vi "Client.vi"() -> ()   [LabVIEW 2009]
panel:
  in  "Example:":string(combo)
  out "time":string
  out "TCP_F":bool
  in  "Exit":bool
  out "IP-status":string
  in  "IP-address":string="10.3.1.41"
  in  "Result?":bool
  in  "Result":string
  in  "Status?":bool
  in  "Status":string
  in  "Send":bool
  in  "CMD":string="Set_PJVS"
  out "TCP_T":bool caption="Status TCP connection"
  out "connection ID":refnum<k5>
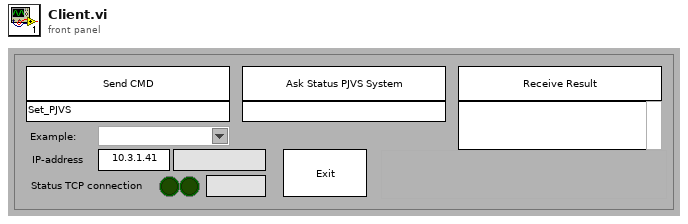
[diagram p1: front panel]
types:
  T1 = enum32{"invalid app kind", "Development System", "Run Time System", "Student Edition", "Embedded LabVIEW", "Evaluation", "Custom"}
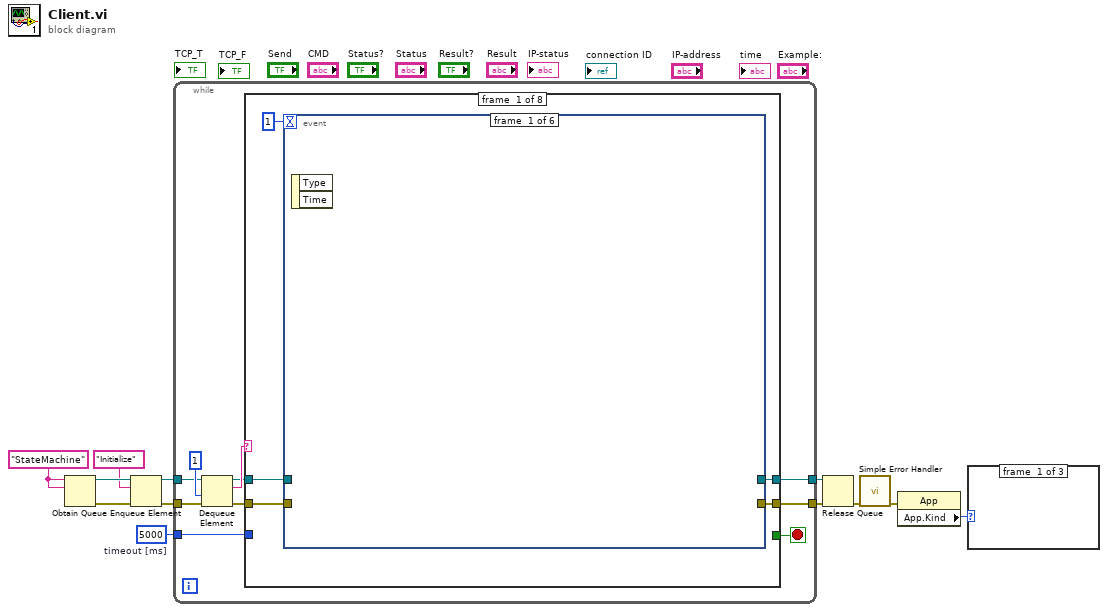
[diagram p0: block diagram]
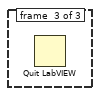
[diagram p3: hidden frame]
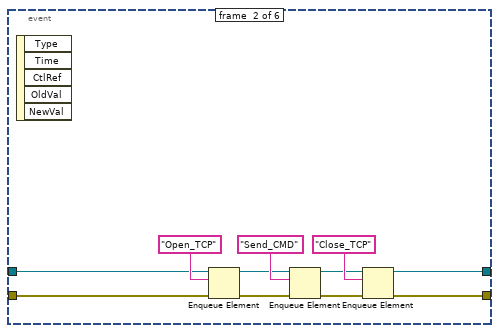
[diagram p4: hidden frame]
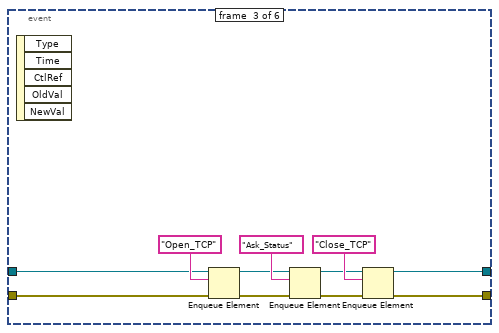
[diagram p5: hidden frame]
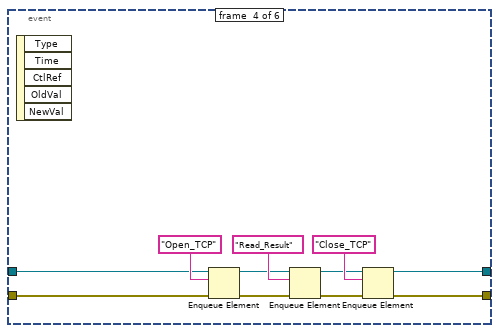
[diagram p6: hidden frame]
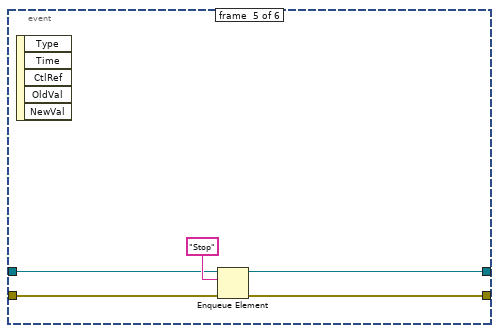
[diagram p7: hidden frame]
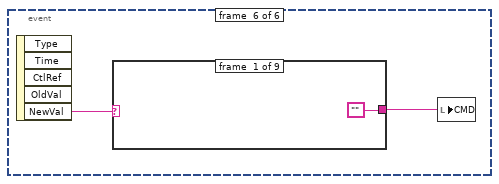
[diagram p8: hidden frame]
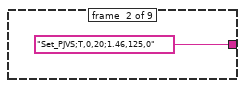
[diagram p9: hidden frame]
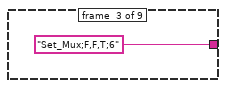
[diagram p10: hidden frame]
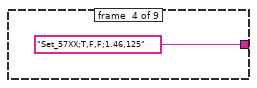
[diagram p11: hidden frame]
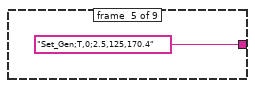
[diagram p12: hidden frame]
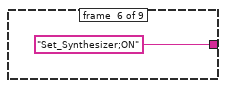
[diagram p13: hidden frame]
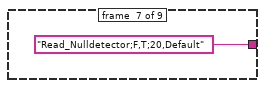
[diagram p14: hidden frame]
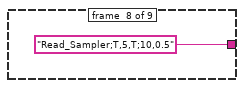
[diagram p15: hidden frame]
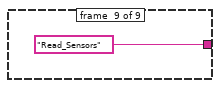
[diagram p16: hidden frame]
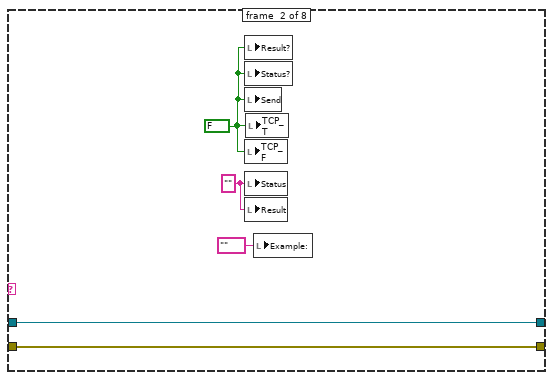
[diagram p17: hidden frame]
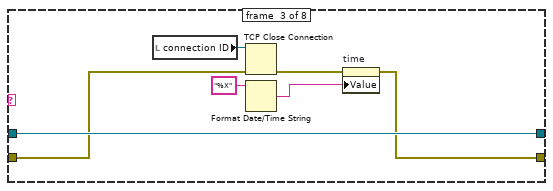
[diagram p18: hidden frame]
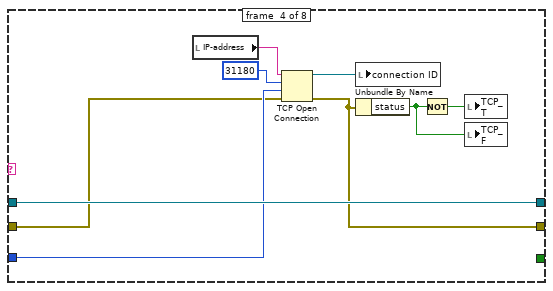
[diagram p19: hidden frame]
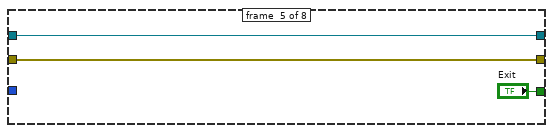
[diagram p20: hidden frame]
diagram:
  w2 = 5000  # timeout [ms]
  w9 = "StateMachine" ("element")
  n1 = Obtain Queue(name (unnamed)=w9, element data type=w9) -> (queue out=w12:refnum<queue>, error out=w11:errorcluster)  [unwired: 3 in, 1 out]
  n2 = Enqueue Element(queue=w12, element="Initialize", error in (no error)=w11) -> (queue out=w8:refnum<queue>, error out=w7:errorcluster)  [unwired: 1 in, 1 out]
  n3 = while {
    tunnel: w8 -> [w21]
    tunnel: w7 -> [w20]
    tunnel: [w18] -> w3
    tunnel: w2 -> [w15]
    tunnel: [w14] -> w1
    stop <- w13 stop-if-true
    n4 = Dequeue Element(queue=w21, timeout in ms (-1)=1, error in (no error)=w20) -> (queue out=w17:refnum<queue>, element=w19:string, error out=w16:errorcluster)  [unwired: 1 out]
    n5 = case shown="\"Read_Result\"" w19 {
      tunnel: [w24 w81 w88 w97 w100 w126 w148 w170] -> w18
      tunnel: w17 -> [w26 w81 w88 w97 w100 w126 w148 w170]
      tunnel: w16 -> [w25 w80 w86 w93 w98 w118 w144 w166]
      tunnel: w15 -> [_ _ _ w94 _ w108 w140 w162]
      tunnel: [w23 w80 w84 w92 w98 w101 w131 w153] -> w14
      tunnel: [_ _ _ _ "Exit" _ _ _] -> w13
      frame #0 {
        n6 = event shown="[5] \"Example:\": Value Change" {
          selector: _ -> [_ _ _ _ _ _]
          dyn-events: _ -> [_ _ _ _ _ _]
          timeout: 1 -> [_ _ _ _ _ _]
          tunnel: w26 -> [_ w31 w42 w53 w62 _]
          tunnel: w25 -> [_ w32 w43 w54 w61 _]
          tunnel: [_ w28 w39 w50 w64 _] -> w24
          tunnel: [_ w33 w44 w55 w63 _] -> w23
          event #0 {
            n7 = event-data() -> ()  [unwired: 1 in, 2 out]
          }
          event #1 {
            n8 = event-data() -> ()  [unwired: 1 in, 5 out]
            n9 = Enqueue Element(queue=w31, element="Open_TCP", error in (no error)=w32) -> (queue out=w30:refnum<queue>, error out=w35:errorcluster)  [unwired: 1 in, 1 out]
            n10 = Enqueue Element(queue=w30, element="Send_CMD", error in (no error)=w35) -> (queue out=w29:refnum<queue>, error out=w34:errorcluster)  [unwired: 1 in, 1 out]
            n11 = Enqueue Element(queue=w29, element="Close_TCP", error in (no error)=w34) -> (queue out=w28:refnum<queue>, error out=w33:errorcluster)  [unwired: 1 in, 1 out]
          }
          event #2 {
            n12 = event-data() -> ()  [unwired: 1 in, 5 out]
            n13 = Enqueue Element(queue=w42, element="Open_TCP", error in (no error)=w43) -> (queue out=w41:refnum<queue>, error out=w46:errorcluster)  [unwired: 1 in, 1 out]
            n14 = Enqueue Element(queue=w41, element="Ask_Status", error in (no error)=w46) -> (queue out=w40:refnum<queue>, error out=w45:errorcluster)  [unwired: 1 in, 1 out]
            n15 = Enqueue Element(queue=w40, element="Close_TCP", error in (no error)=w45) -> (queue out=w39:refnum<queue>, error out=w44:errorcluster)  [unwired: 1 in, 1 out]
          }
          event #3 {
            n16 = event-data() -> ()  [unwired: 1 in, 5 out]
            n17 = Enqueue Element(queue=w53, element="Open_TCP", error in (no error)=w54) -> (queue out=w52:refnum<queue>, error out=w57:errorcluster)  [unwired: 1 in, 1 out]
            n18 = Enqueue Element(queue=w52, element="Read_Result", error in (no error)=w57) -> (queue out=w51:refnum<queue>, error out=w56:errorcluster)  [unwired: 1 in, 1 out]
            n19 = Enqueue Element(queue=w51, element="Close_TCP", error in (no error)=w56) -> (queue out=w50:refnum<queue>, error out=w55:errorcluster)  [unwired: 1 in, 1 out]
          }
          event #4 {
            n20 = event-data() -> ()  [unwired: 1 in, 5 out]
            n21 = Enqueue Element(queue=w62, element="Stop", error in (no error)=w61) -> (queue out=w64:refnum<queue>, error out=w63:errorcluster)  [unwired: 1 in, 1 out]
          }
          event #5 {
            n22 = event-data() -> ("NewVal"=w67:string)  [unwired: 1 in, 4 out]
            n23 = case shown="\"Read_Sampler\"" w67 {
              tunnel: ["" "Set_PJVS;T,0,20;1.46,125,0" ("NewVal") "Set_Mux;F,F,T;6" ("NewVal") "Set_57XX;T,F,F;1.46,125" ("NewVal") "Set_Gen;T,0;2.5,125,170.4" ("NewVal") "Set_Synthesizer;ON" ("NewVal") "Read_Nulldetector;F,T;20,Default" ("NewVal") "Read_Sampler;T,5,T;10,0.5" ("NewVal") "Read_Sensors" ("NewVal")] -> w66
              frame #0 {
              }
              frame #1 {
              }
              frame #2 {
              }
              frame #3 {
              }
              frame #4 {
              }
              frame #5 {
              }
              frame #6 {
              }
              frame #7 {
              }
              frame #8 {
              }
            }
            n24 = local write "CMD"(w66) -> ()
          }
        }
      }
      frame #1 {
        w79 = "" ("Status")
        w78 = FALSE ("TCP_T")
        n25 = local write "Result?"(w78) -> ()
        n26 = local write "Status?"(w78) -> ()
        n27 = local write "Send"(w78) -> ()
        n28 = local write "TCP_F"(w78) -> ()
        n29 = local write "Status"(w79) -> ()
        n30 = local write "Result"(w79) -> ()
        n31 = local write "TCP_T"(w78) -> ()
        n32 = local write "Example:"("" ("Example:")) -> ()
      }
      frame #2 {
        n33 = local read "connection ID"() -> (w87:refnum<k5>)
        n34 = TCP Close Connection(connection ID=w87, error in (no error)=w86) -> (error out=w85:errorcluster)  [unwired: 1 in, 1 out]
        n35 = Format Date/Time String(time format string (%c)="%X") -> (date/time string=w83:string)  [unwired: 2 in]
        n36 = property on="time" class="Str"(error in=w85, "Value"=w83) -> (error out=w84:errorcluster)  [unwired: 1 in, 1 out]
      }
      frame #3 {
        n37 = local read "IP-address"() -> (w95:string)
        n38 = TCP Open Connection(address=w95, remote port or service name=u16 31180, timeout ms (60000)=w94, error in (no error)=w93) -> (connection ID=w91:refnum<k5>, error out=w92:errorcluster)  [unwired: 1 in]
        n39 = local write "connection ID"(w91) -> ()
        n40 = Unbundle By Name(w92) -> ("status"=w89:bool)
        n41 = Not(x=w89) -> (.not. x?=w90:bool)
        n42 = local write "TCP_T"(w90) -> ()
        n43 = local write "TCP_F"(w89) -> ()
      }
      frame #4 {
      }
      frame #5 {
        n44 = local read "connection ID"() -> (w121:refnum<k5>)
        n45 = local read "CMD"() -> (w105:string)
        n46 = String Length(string=w105) -> (length=w107:i32)
        n47 = Number To Decimal String(number=u8 1) -> (decimal integer string=w125:string)  [unwired: 1 in]
        n48 = To Unsigned Word Integer(number=w107) -> (unsigned 16bit integer=w104:u16)
        n49 = TCP Write(connection ID=w121, data in=w125, error in (no error)=w118, 9:w108) -> (connection ID out=w122:refnum<k5>, error out=w123:errorcluster)  [unwired: 1 out]
        n50 = Type Cast(type=w105, x=w104) -> (*(type *) &x=w106:string)
        n51 = TCP Write(connection ID=w122, data in=w106, error in (no error)=w123, 9:w108) -> (connection ID out=w120:refnum<k5>, error out=w119:errorcluster)  [unwired: 1 out]
        n52 = TCP Write(connection ID=w120, data in=w105, error in (no error)=w119, 9:w108) -> (connection ID out=w110:refnum<k5>, error out=w109:errorcluster)  [unwired: 1 out]
        n53 = TCP Read(connection ID=w110, bytes to read=2, error in (no error)=w109, 9:w108) -> (data out=w116:string, error out=w101:errorcluster)  [unwired: 1 in, 1 out]
        n54 = Equal?(x="OK", y=w116) -> (x = y?=w114:bool)
        n55 = stacked-sequence {
          tunnel: w101 -> [_]
          frame #0 {
            n56 = property on="Send" class="Bool (strict)"("Value"=FALSE ("Send")) -> ()  [unwired: 2 in, 2 out]
          }
        }
        n57 = Unbundle By Name(w101) -> ("status"=w102:bool)
        n58 = Select(t="transmitted" ("x"), s=w114, f="error" ("x")) -> (s? t:f=w111:string)
        n59 = local write "IP-status"(w111) -> ()
        n60 = Not(x=w102) -> (.not. x?=w103:bool)
        n61 = local write "TCP_F"(w102) -> ()
        n62 = local write "TCP_T"(w103) -> ()
      }
      frame #6 {
        n63 = local read "connection ID"() -> (w145:refnum<k5>)
        n64 = Number To Decimal String(number=3) -> (decimal integer string=w147:string)  [unwired: 1 in]
        n65 = TCP Write(connection ID=w145, data in=w147, error in (no error)=w144, 9:w140) -> (connection ID out=w142:refnum<k5>, error out=w143:errorcluster)  [unwired: 1 out]
        n66 = TCP Read(connection ID=w142, bytes to read=2, error in (no error)=w143, 9:w140) -> (connection ID out=w141:refnum<k5>, data out=w134:string, error out=w139:errorcluster)  [unwired: 1 in]
        n67 = Type Cast(type=u16 0 ("bytes to read"), x=w134) -> (*(type *) &x=w135:u16)
        n68 = To Long Integer(number=w135) -> (32bit integer=w133:i32)
        n69 = TCP Read(connection ID=w141, bytes to read=w133, error in (no error)=w139, 9:w140) -> (data out=w138:string, error out=w128:errorcluster)  [unwired: 1 in, 1 out]
        n70 = local write "Status"(w138) -> ()
        n71 = property on="IP-status" class="Str"(error in=w128, "Value"="received" ("IP-status")) -> (error out=w131:errorcluster)  [unwired: 1 in, 1 out]
        n72 = Unbundle By Name(w128) -> ("status"=w129:bool)
        n73 = stacked-sequence {
          tunnel: w131 -> [_]
          frame #0 {
            n74 = property on="Status?" class="Bool (strict)"("Value"=FALSE ("Send")) -> ()  [unwired: 2 in, 2 out]
          }
        }
        n75 = Not(x=w129) -> (.not. x?=w130:bool)
        n76 = local write "TCP_F"(w129) -> ()
        n77 = local write "TCP_T"(w130) -> ()
      }
      frame #7 {
        n78 = local read "connection ID"() -> (w167:refnum<k5>)
        n79 = Number To Decimal String(number=2) -> (decimal integer string=w169:string)  [unwired: 1 in]
        n80 = TCP Write(connection ID=w167, data in=w169, error in (no error)=w166, 9:w162) -> (connection ID out=w164:refnum<k5>, error out=w165:errorcluster)  [unwired: 1 out]
        n81 = TCP Read(connection ID=w164, bytes to read=4, error in (no error)=w165, 9:w162) -> (connection ID out=w163:refnum<k5>, data out=w156:string, error out=w161:errorcluster)  [unwired: 1 in]
        n82 = Type Cast(type=u32 0 ("bytes to read"), x=w156) -> (*(type *) &x=w157:u32)
        n83 = To Unsigned Long Integer(number=w157) -> (unsigned 32bit integer=w155:u32)
        n84 = TCP Read(connection ID=w163, bytes to read=w155, error in (no error)=w161, 9:w162) -> (data out=w160:string, error out=w150:errorcluster)  [unwired: 1 in, 1 out]
        n85 = local write "Result"(w160) -> ()
        n86 = Unbundle By Name(w150) -> ("status"=w151:bool)
        n87 = property on="IP-status" class="Str"(error in=w150, "Value"="received" ("IP-status")) -> (error out=w153:errorcluster)  [unwired: 1 in, 1 out]
        n88 = stacked-sequence {
          tunnel: w153 -> [_]
          frame #0 {
            n89 = property on="Result?" class="Bool (strict)"("Value"=FALSE ("Status?")) -> ()  [unwired: 2 in, 2 out]
          }
        }
        n90 = Not(x=w151) -> (.not. x?=w152:bool)
        n91 = local write "TCP_F"(w151) -> ()
        n92 = local write "TCP_T"(w152) -> ()
      }
    }
  }
  n93 = Release Queue(queue=w3, error in (no error)=w1) -> (error out=w4:errorcluster)  [unwired: 1 in, 2 out]
  n94 = call <vilib>:"Simple Error Handler.vi"("error in (no error)"=w4) -> ("error out"=w6:errorcluster)  [unwired: 4 in, 4 out]
  n95 = property class="App"(error in=w6) -> ("App.Kind"=w5:T1)  [unwired: 1 in, 2 out]
  n96 = case shown="\"Run Time System\"" w5 {
    frame #0 {
    }
    frame #1 {
    }
    frame #2 {
      n97 = Quit LabVIEW() -> ()  [unwired: 1 in]
    }
  }
